vi "python_acquisition_multiple_in_python.vi"(0 "MH_UIThread_Data":T1={"Init Info"={"Library Version"="", "Serial No."="", "Model"="", "Partnum"="", "Version"="", "features"=0, "nchannels"=0, "Base Resolution"=0.0, "Bin Steps"=0}, "DevIdx"=0, "SyncDivider"=1, "SyncOffset"=0, "SyncLevel"=50, "Channels"=[], "CurrentChannels"=[], "AcqTime"=1, "Binning"=1, "HistoOffset"=1, "HistoLen"=1024, "StopOvl."=FALSE, "OvlLevel"=1024, "SyncEdge"=1, "StartMeas"=FALSE, "HistoLength"=0, "Resolution"=0.0, "Run cont."=FALSE, "Status"="", "SyncRate"=0, "BitShift"=0, "HistoAcqTime"=0.0, "SyncRateStart"=0, "UseDeadTime"=FALSE, "SyncDeadTime"=800, "SetInpChan"=[], "max value"=[], "CoincidenceArray"=[], "Instr Enqueuers"={"MH Enqueuer"=refnum, "KIM Enqueuer"=refnum}, "Histo On"=FALSE} {"SyncDeadTime" min=800 max=160000 step=1; "SyncEdge" items=["falling", "rising"]; "SyncDivider" items=["1", "2", "4", "8", "16"]; "SyncOffset" min=0 max=100000 step=1; "SyncLevel" min=0 max=800 step=1; "AcqTime" min=1 max=360000 step=1; "Binning" items=["1", "2", "4", "8", "16", "32", "64", "128", "256", "512", "1024", "2048", "4096", "8192", "16384", "32768", "65536", "131072", "262144", "524288", "1048576", "2097152", "4194304", "8388608", "16777216", "3355443225"]; "HistoOffset" min=0 max=500 step=1; "HistoLen" min=1024 max=65536 step=1024; "Channels"."DeadTime" min=800 max=160000 step=1; "Channels"."Edge" items=["falling", "rising"]; "Channels"."Offset" min=-100000 max=100000 step=10; "Channels"."Level" min=-1200 max=1200 step=1}, 1 "FileName":string, 2 "mode":i32=2, 3 "Number \nof Acquisitions":i32, 4 "Directory":string) -> (7 "error out":errorcluster)   [LabVIEW 2023]
uses:
  Types/MH_InputChannel.ctl
  Types/MH_SetInpChanCmds.ctl
  Types/MH_SetInpChanData.ctl
  Types/MH_UIThread_Data_T2.ctl
  _lib/PQ/MultiHarp/MH_InitInfo.ctl
  typedefs/typedefs.lvlib
  <vilib>/ActorFramework/Message Enqueuer/Message Enqueuer.lvclass
panel:
  out "return value":i32
  # "Sync"
  # "Histogram"
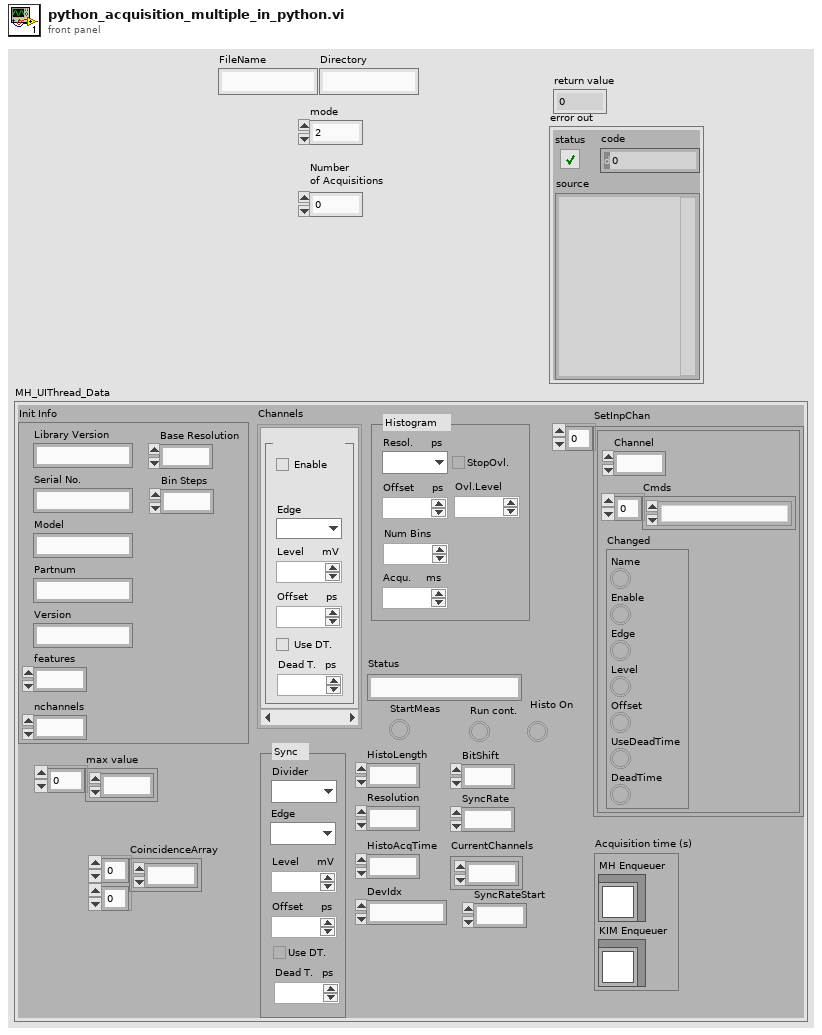
[diagram p1: front panel]
types:
  T1 = typedef "MH_UIThread_Data_T2.ctl" = cluster{"Init Info":T2, "DevIdx":i32, "SyncDivider":i32, "SyncOffset":i32, "SyncLevel":i32, "Channels":T3[], "CurrentChannels":i32[], "AcqTime":i32, "Binning":i32, "HistoOffset":i32, "HistoLen":i32, "StopOvl.":bool, "OvlLevel":u32, "SyncEdge":i32, "StartMeas":bool, "HistoLength":i32, "Resolution":dbl, "Run cont.":bool, "Status":string, "SyncRate":i32, "BitShift":i32, "HistoAcqTime":dbl, "SyncRateStart":i32, "UseDeadTime":bool, "SyncDeadTime":i32, "SetInpChan":T4[], "max value":u32[], "CoincidenceArray":dbl[][], "Instr Enqueuers":cluster{"MH Enqueuer":refnum<class "Message Enqueuer.lvclass">, "KIM Enqueuer":refnum<class "Message Enqueuer.lvclass">}, "Histo On":bool}
  T2 = typedef "typedefs.lvlib/MH_InitInfo.ctl" = cluster{"Library Version":string, "Serial No.":string, "Model":string, "Partnum":string, "Version":string, "features":i32, "nchannels":i32, "Base Resolution":dbl, "Bin Steps":i32}
  T3 = typedef "MH_InputChannel.ctl" = cluster{"Name":string, "Enable":bool, "Edge":i32, "Level":i32, "Offset":i32, "UseDeadTime":bool, "DeadTime":i32}
  T4 = typedef "MH_SetInpChanData.ctl" = cluster{"Channel":i32, "Cmds":T5[], "Changed":cluster{"Name":bool, "Enable":bool, "Edge":bool, "Level":bool, "Offset":bool, "UseDeadTime":bool, "DeadTime":bool}}
  T5 = typedef "MH_SetInpChanCmds.ctl" = enum16{"SetInpChanEnable", "SetInpChanOffset", "SetInpChanDeadTime", "SetInpChanTrg"}
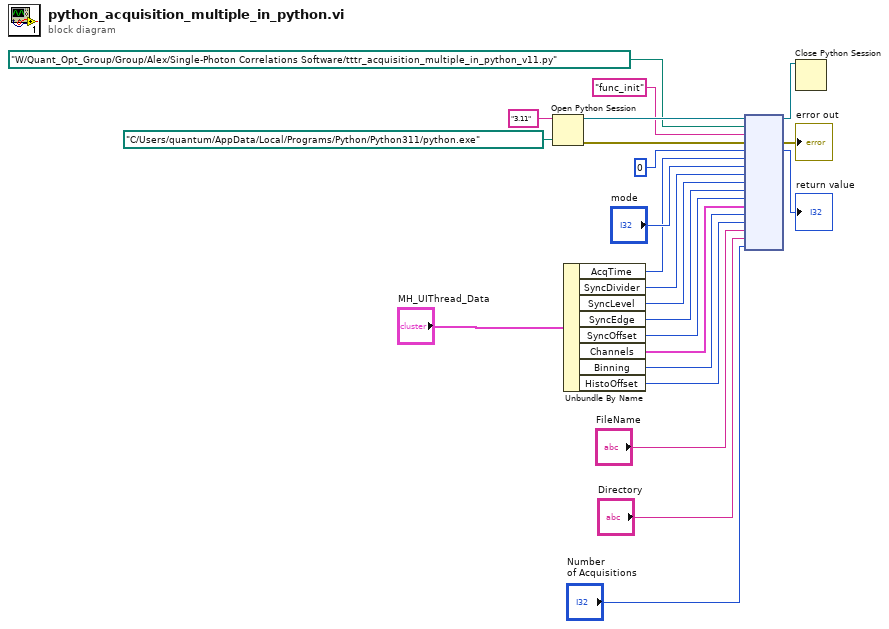
[diagram p0: block diagram]
diagram:
  n1 = Open Python Session(python version="3.11" ("Python version"), python path=path "C:/Users/quantum/AppData/Local/Programs/Python/Python311/python.exe" ("Python path")) -> (session out=w23:refnum<k35>, error out=w21:errorcluster)  [unwired: 1 in]
  n2 = Unbundle By Name("MH_UIThread_Data") -> ("AcqTime"=w10:i32, "SyncDivider"=w9:i32, "SyncLevel"=w8:i32, "SyncEdge"=w7:i32, "SyncOffset"=w6:i32, "Channels"=w5:T3[], "Binning"=w4:i32, "HistoOffset"=w3:i32)
  n3 = node(w23, path "W:/Quant_Opt_Group/Group/Alex/Single-Photon Correlations Software/tttr_acquisition_multiple_in_python_v11.py" ("module path"), "func_init" ("function name"), w21, 0, w10, "mode", w9, w8, w7, w6, w5, w4, w3, "FileName", "Directory", "Number \nof Acquisitions") -> (w22:refnum<k35>, →"error out":errorcluster, →"return value":i32)  [unwired: 12 in, 2 out]
  n4 = Close Python Session(session in=w22) -> ()  [unwired: 1 in, 1 out]
